vi "Write Path in.vi"(8 "error in (no error)":errorcluster, 10 "Path in":string, 11 "[Test Case] Fix Path in":refnum<class "[Test Case] Fix path.lvclass">=refnum) -> (0 "error out":errorcluster, 3 "[Test Case] Fix Path out":refnum<class "[Test Case] Fix path.lvclass">)   [LabVIEW 2016, in "Tests.lvlib" / "[Test Case] Fix path.lvclass"]
uses:
  [Test Case] Fix path.lvclass
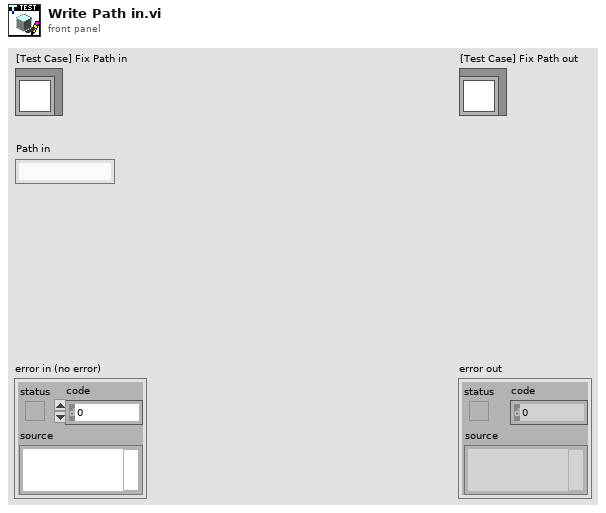
[diagram p1: front panel]
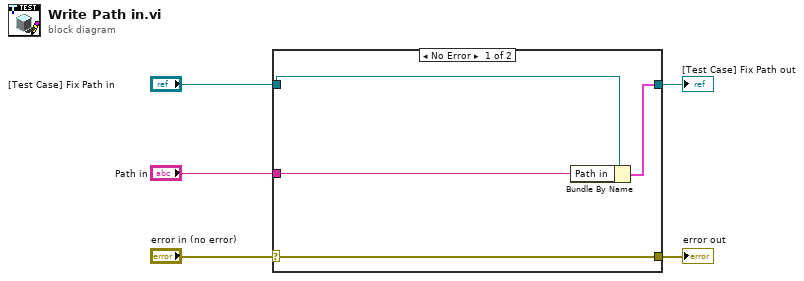
[diagram p0: block diagram]
diagram:
  n1 = case shown="No Error" "error in (no error)" {
    selector: "error in (no error)" -> [w9 w10]
    tunnel: [w9 w10] -> w4
    tunnel: [w7 w11] -> w2
    tunnel: "[Test Case] Fix Path in" -> [w8 w11]
    tunnel: "Path in" -> [w6 _]
    frame No Error {
      n2 = Bundle By Name(cluster=w8, "Path in"=w6) -> (w7:cluster{})
    }
    frame Error {
    }
  }
  "error out" <- w4
  "[Test Case] Fix Path out" <- w2
